vi "Icon_Set Vi Icon.vi"(8 "Error":errorcluster, 9 "Image Cluster":T1, 11 "VI REF":refnum<vi>) -> (0 "Error Out":errorcluster, 3 "VI REF Out":refnum<vi>)   [LabVIEW 2009]
doc: "Set the new icon data with Image data"
uses:
  Controls/Cluster/Cluster_Image Data.ctl
  Controls/Cluster/CLuster_Selectoin Box.ctl
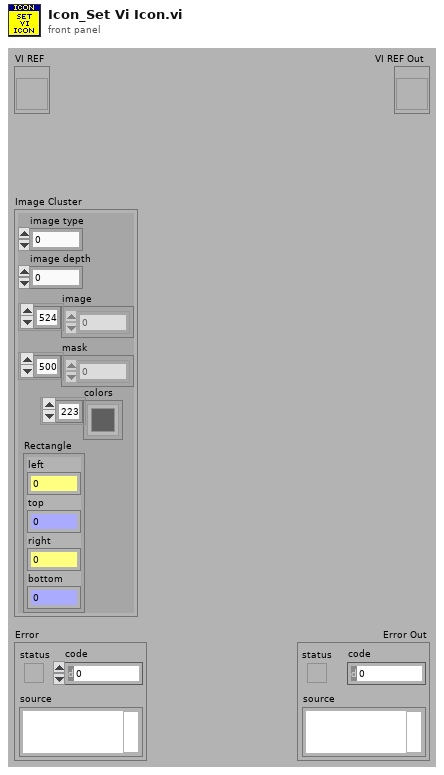
[diagram p1: front panel]
types:
  T1 = typedef "Cluster_Image Data.ctl" = cluster{"image type":i32, "image depth":i32, "image":u8[], "mask":u8[], "colors":u32[], "Rectangle":T2}
  T2 = typedef "CLuster_Selectoin Box.ctl" = cluster{"left":i16, "top":i16, "right":i16, "bottom":i16}
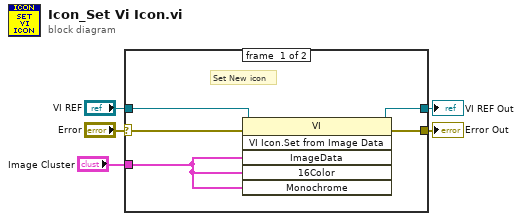
[diagram p0: block diagram]
diagram:
  n1 = case shown="No Error" "Error" {
    selector: "Error" -> [w7 w11]
    tunnel: "VI REF" -> [w10 w12]
    tunnel: [w9 w12] -> w4
    tunnel: [w8 w11] -> w3
    tunnel: "Image Cluster" -> [w6 _]
    frame #0 {
      # "Set New icon"
      n2 = invoke class="VI" method="VI Icon.Set from Image Data"(reference=w10, error in=w7, "ImageData"=w6, "16Color"=w6, "Monochrome"=w6) -> (reference out=w9:refnum<vi>, error out=w8:errorcluster)  [unwired: 1 in, 4 out]
    }
    frame #1 {
    }
  }
  "VI REF Out" <- w4
  "Error Out" <- w3
